vi "Write Configuration Settings File.vi"() -> ()   [LabVIEW 2015]
doc: "Illustrates how to create and write a configuration settings file.\n\nInstructions:\nEnter values in the controls on the front panel then click on the Run Arrow.\nTo read the file, run Read Configuration Settings File.vi located in the file\\config.llb."
uses:
  Boiler System Globals.vi
  <vilib>/Utility/config.llb/Write Key (Double).vi
  <vilib>/Utility/config.llb/Write Key (U32).vi
  <vilib>/Utility/config.llb/NI_LVConfig.lvlib
panel:
  in  "Pilot Decrement (ms)":u32=50
  in  "Pilot Increment (ms)":u32=100
  in  "Flame Threshold":u32=30
  in  "Purge Time":u32=2
  in  "Fuel Control Valve Minimum":dbl=10.0
  in  "Fuel Control Valve Maximum":dbl=75.0
  # "Instructions:\nEnter values in the controls below, then click on the Run arrow.  The VI will write these values into the selected configuration settings file."
  # "MHL"
  # "Controller"
  # "Boiler"
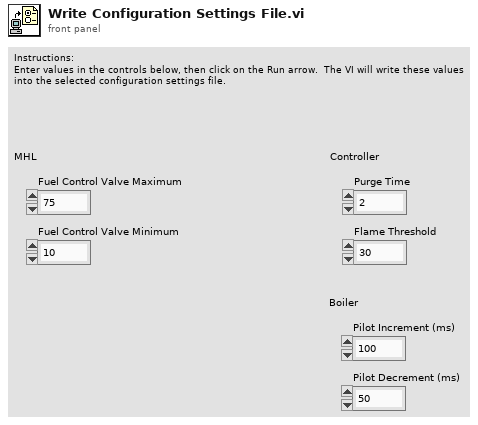
[diagram p1: front panel]
types:
  T1 = typedef "NI_LVConfig.lvlib/Config Data RefNum.ctl" = refnum<k1>
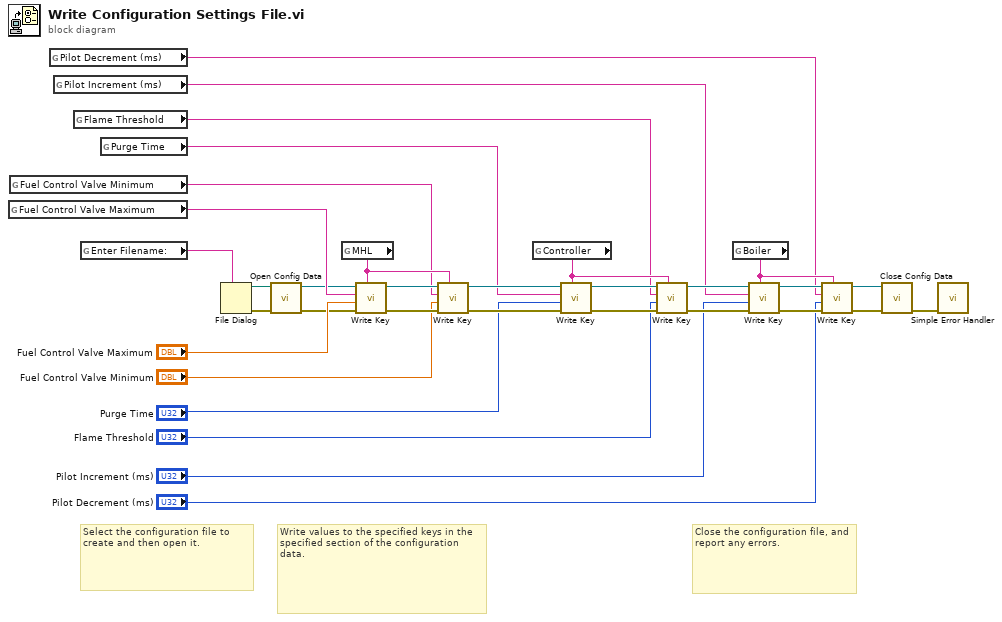
[diagram p0: block diagram]
diagram:
  # "Close the configuration file, and report any errors."
  # "Write values to the specified keys in the specified section of the configuration data."
  # "Select the configuration file to create and then open it."
  n1 = global read "Boiler System Globals.vi" "Fuel Control Valve Maximum"() -> (w29:string)
  n2 = global read "Boiler System Globals.vi" "Fuel Control Valve Minimum"() -> (w20:string)
  n3 = global read "Boiler System Globals.vi" "Pilot Decrement (ms)"() -> (w2:string)
  n4 = global read "Boiler System Globals.vi" "Pilot Increment (ms)"() -> (w3:string)
  n5 = global read "Boiler System Globals.vi" "Flame Threshold"() -> (w12:string)
  n6 = global read "Boiler System Globals.vi" "Enter Filename:"() -> (w31:string)
  n7 = global read "Boiler System Globals.vi" "Purge Time"() -> (w17:string)
  n8 = File Dialog(7:w31) -> (0:w30:errorcluster, 3:w33:path)  [unwired: 1 in, 7 out]
  n9 = call <vilib>:"Open Config Data.vi"("error in (no error)"=w30, "configuration file path"=w33) -> ("error out"=w26:errorcluster, "refnum"=w27:T1)  [unwired: 1 in, 7 out]
  n10 = global read "Boiler System Globals.vi" "MHL"() -> (w23:string)
  n11 = call-poly <vilib>:"Write Key.vi"("section"=w23, "error in (no error)"=w26, "value"="Fuel Control Valve Maximum", "key"=w29, "refnum"=w27) -> ("error out"=w25:errorcluster, "refnum out"=w24:T1)  [unwired: 4 in, 1 out]
  n12 = call-poly <vilib>:"Write Key.vi"("section"=w23, "error in (no error)"=w25, "value"="Fuel Control Valve Minimum", "key"=w20, "refnum"=w24) -> ("error out"=w22:errorcluster, "refnum out"=w18:T1)  [unwired: 4 in, 1 out]
  n13 = global read "Boiler System Globals.vi" "Controller"() -> (w14:string)
  n14 = call-poly <vilib>:"Write Key.vi"("section"=w14, "error in (no error)"=w22, "value"="Purge Time", "key"=w17, "refnum"=w18) -> ("error out"=w19:errorcluster, "refnum out"=w15:T1)  [unwired: 4 in, 1 out]
  n15 = call-poly <vilib>:"Write Key.vi"("section"=w14, "error in (no error)"=w19, "value"="Flame Threshold", "key"=w12, "refnum"=w15) -> ("error out"=w8:errorcluster, "refnum out"=w7:T1)  [unwired: 4 in, 1 out]
  n16 = global read "Boiler System Globals.vi" "Boiler"() -> (w11:string)
  n17 = call-poly <vilib>:"Write Key.vi"("section"=w11, "error in (no error)"=w8, "value"="Pilot Increment (ms)", "key"=w3, "refnum"=w7) -> ("error out"=w9:errorcluster, "refnum out"=w10:T1)  [unwired: 4 in, 1 out]
  n18 = call-poly <vilib>:"Write Key.vi"("section"=w11, "error in (no error)"=w9, "value"="Pilot Decrement (ms)", "key"=w2, "refnum"=w10) -> ("error out"=w5:errorcluster, "refnum out"=w6:T1)  [unwired: 4 in, 1 out]
  n19 = call <vilib>:"Close Config Data.vi"("error in (no error)"=w5, "refnum"=w6) -> ("error out"=w32:errorcluster)  [unwired: 1 in, 8 out]
  n20 = call <vilib>:"Simple Error Handler.vi"("error in (no error)"=w32) -> ()  [unwired: 1 in, 8 out]
